vi "Emballage_BDD_Identification_Vdll.vi"(5 "Glissière":refnum<vi>, 6 "lecture seul possible ?":bool, 8 "error in":errorcluster caption="entrée d'erreur", 9 "Posage choisi":string="S112.1229", 11 "chemin connexion complet":path=path "U:/MTD_PRD_TESTS/PARAM_TESTS/PROD_Data-Admin/Support_FAS/Connexion_BDD_VSX.udl") -> (0 "error Out":errorcluster caption="error OUT", 1 "Employe selectionne":T1={"ID Employe"="885", "NOM "="MARTIN SEBASTIEN", "Code ID Employe"="0f00b6435b", "abreviation"="SMA"}, 2 "OK":bool, 3 "lecture seul":bool, 7 "Annulé":bool)   [LabVIEW 2020]
doc: "Vi qui identifie l'utilisateur. Ensuite il vérifie qu'il a ouvert une gamme de travail et finalement qu'il a les accès nécessaire pour ce travail."
uses:
  <vilib>/Utility/error.llb/DialogType.ctl
  Modules/FS/60_FS_Controles/60_FS_SetGet.ctl
panel:
  out "Glissière 2":u8(slide)=100 caption="Identification terminé." scale=0.0..100.0
  out "Table":string[][](table)=[["Nom", "Abréviation", "code", "code bar", "Saisi des H", "Responsable", "S112.1108b", "S112.1065", "S112.1066", "S121.0017", "S122.0009", "Flatprop", "Emballage", "S112.1229/S112.1254", "S112.1289", "S002.0002"], ["YURDAKUL ARZU", "AYU", "AYU_FAS", "0f00b69799", "0", "0", "0", "0", "0", "0", "0", "0", "0", "", "", ""], ["DEDERDING BRIGITTE", "BDE", "BDE_FAS", "0f00b64582", "1", "resp", "1", "1", "1", "1", "1", "1", "1", "1", "1", "1"], ["DA FONSECA CARLOS MANUEL", "CDA", "CDA_FAS", "0f00b64d63", "1", "resp", "1", "1", "1", "1", "1", "1", "1", "1", "1", "1"], ["DOS ANJOS MARIA  CRISTINA", "MDO", "MDO_FAS", "0f00dfc69b", "1", "0", "1", "1", "1", "1", "1", "1", "1", "1", "1", "1"], ["BIANCANIELLO MARIE-JOSE", "MJB", "MJB_FAS", "0f00b65673", "1", "0", "0", "0", "0", "0", "0", "0", "1", "", "", ""], ["DERIVAZ PASCAL", "PDE", "PDE_FAS", "0f00b64c64", "0", "resp", "1", "1", "1", "1", "1", "1", "1", "1", "1", "1"], ["CRAUSAZ-DEMIRTAS SERAP", "SCR", "SCR_FAS", "0f00b64e53", "1", "0", "0", "1", "1", "1", "1", "1", "1", "", "", ""], ["GILLIERON  SABINE", "SLE", "SLE_FAS", "0f00b62fc0", "1", "0", "0", "1", "1", "1", "1", "0", "1", "", "", ""], ["MARTIN SEBASTIEN", "SMA", "SMA_FAS", "0f00b6435b", "1", "resp", "1", "1", "1", "1", "1", "1", "1", "1", "1", "1"], ["VUONG VAN-THANH", "VVT", "VVT_FAS", "0f00b6a8bc", "1", "0", "0", "0", "0", "0", "0", "0", "1", "", "", ""], ["PEREIRA CARLA SOFIA", "PCR", "PCR_FAS", "0f00dfcec4", "1", "0", "0", "0", "0", "0", "0", "1", "1", "", "", ""], ["SANTOS ARMINDA", "ASA", "ASA_FAS", "0f00dfded8", "1", "0", "0", "1", "1", "0", "0", "0", "1", "", "", ""], ["AMANAKO KIBEYA", "KAM", "KAM_FAS", "0f00b6461f", "1", "0", "0", "0", "0", "0", "0", "0", "1", "", "", ""], ["PICOT BRUNO", "BPI", "BPI_FAS", "", "0", "resp", "0", "0", "0", "0", "0", "1", "1", "", "", ""], ["inconnu", "ACK", "ACK_FAS", "inconnu", "0", "resp", "0", "0", "0", "0", "0", "1", "1", "", "", ""], ["FRANCISCO HELIA", "HFR", "HFR_FAS", "0f00ff3428", "1", "0", "0", "1", "1", "0", "0", "0", "1", "", "", ""], ["BERTHOLET MAGALI", "MBE", "MBE_FAS", "0f00debcbf", "1", "0", "0", "0", "0", "0", "0", "1", "1", "", "", ""], ["BEN AYAD DIECKMANN LATIFA", "LBA", "LBA_FAS", "0f00ff602d", "1", "0", "0", "0", "0", "0", "0", "0", "1", "", "", ""], ["ROBERT FABIEN", "FAR", "FAR_FAS", "0f00b648bf", "1", "0", "0", "0", "0", "0", "0", "1", "1", "", "", ""], ["GABRIEL CASSAB SUSANA", "SUG", "SUG_FAS", "0f00b65355", "1", "0", "0", "0", "0", "0", "0", "0", "1", "", "", ""], ["BOURAOUI MOURAD", "MBU", "MBU_FAS", "", "0", "resp", "0", "0", "0", "0", "0", "0", "0", "", "", ""], ["BIGLER ORNELLA", "OBI", "OBI_FAS", "0f00b651a2", "1", "0", "1", "1", "1", "1", "1", "0", "1", "1", "1", "1"], ["BRISSONNETTE MIRELLA", "MBI", "MBI_FAS", "0f00e3ba9c", "1", "0", "0", "0", "0", "0", "0", "1", "1", "", "", ""], ["MARTINS ELISA", "ELM", "ELM_FAS", "0f00debd53", "1", "0", "0", "0", "0", "0", "0", "0", "1", "1", "", ""], ["JEANDENANT PASCALE", "PJE", "PJE_FAS", "0f00ff2670", "1", "0", "0", "0", "0", "0", "0", "0", "1", "", "", ""], ["NECHYTAYLO DARYNA", "DNE", "DNE_FAS", "0f00ff68ed", "1", "0", "0", "0", "0", "0", "0", "1", "1", "", "", ""], ["SILVA MONTEIRO DULCELINA", "DSI", "DSI_FAS", "0f00ff4204", "1", "0", "0", "0", "0", "0", "0", "1", "1", "", "", ""], ["PAHUD ELIANE", "EPU", "EPA_FAS", "0f00ff65d6", "1", "0", "0", "0", "0", "0", "0", "1", "1", "", "", ""], ["THOMASSIN CATHERINE", "TCA", "TCA_FAS", "0f00ff696c", "1", "resp", "0", "0", "0", "0", "0", "0", "0", "1", "1", "1"], ["SIMOND DANIELE", "SDA", "SDA_FAS", "0f00ff2ff9", "1", "0", "0", "0", "0", "0", "0", "0", "0", "", "", ""], ["HORTER VALERIE", "VHO", "VHO_FAS", "0f00ff1ecc", "1", "0", "0", "0", "0", "0", "0", "1", "1", "", "", ""], ["CHENAL JEROME", "JCH", "JCH_FAS", "0f00f6d812", "0", "0", "0", "0", "0", "0", "0", "0", "0", "", "", ""], ["BEN AYAD DIECKMANN LATIFA", "LBA", "LBA_FAS", "0f00ff602d", "1", "0", "0", "0", "0", "0", "0", "0", "0", "", "", ""], ["ANTUNES CARLA MARIA", "CAN", "CAN_FAS", "0f00f76887", "1", "0", "0", "0", "0", "0", "0", "0", "0", "", "", ""], ["DEMIRALMAZ SEMRA", "SDM", "SDM_FAS", "0f00ff42a4", "1", "0", "0", "0", "0", "0", "0", "0", "0", "", "", ""], ["DESARZENS MARIANNE", "MDN", "MDN_FAS", "0f00f6e3b5", "1", "0", "0", "0", "0", "0", "0", "0", "0", "", "", ""], ["inconnu", "HRO", "HRO_FAS", "inconnu", "0", "0", "0", "0", "0", "0", "0", "0", "0", "", "", ""], ["SEMEDO SANCHES MARIA FATIMA", "MSM", "MSM_FAS", "0f00f767ff", "1", "0", "0", "0", "0", "0", "0", "1", "1", "", "", ""], ["inconnu", "PHG", "PHG_FAS", "inconnu", "1", "resp", "1", "1", "1", "1", "1", "1", "1", "1", "1", "1"], ["GUIDEZ LIONEL", "LGU", "LGU_FAS", "0f00f6cad9", "1", "resp", "1", "1", "1", "1", "1", "1", "1", "1", "1", "1"], ["NEVEU CELINE", "CNE", "CNE_FAS", "0f00ff1822", "1", "0", "0", "0", "0", "0", "0", "1", "1", "", "", ""], ["AISSAOUI SAOUSSEN", "SAI", "SAI_FAS", "0f00ff4123", "1", "0", "0", "0", "0", "0", "0", "1", "1", "", "", ""]]
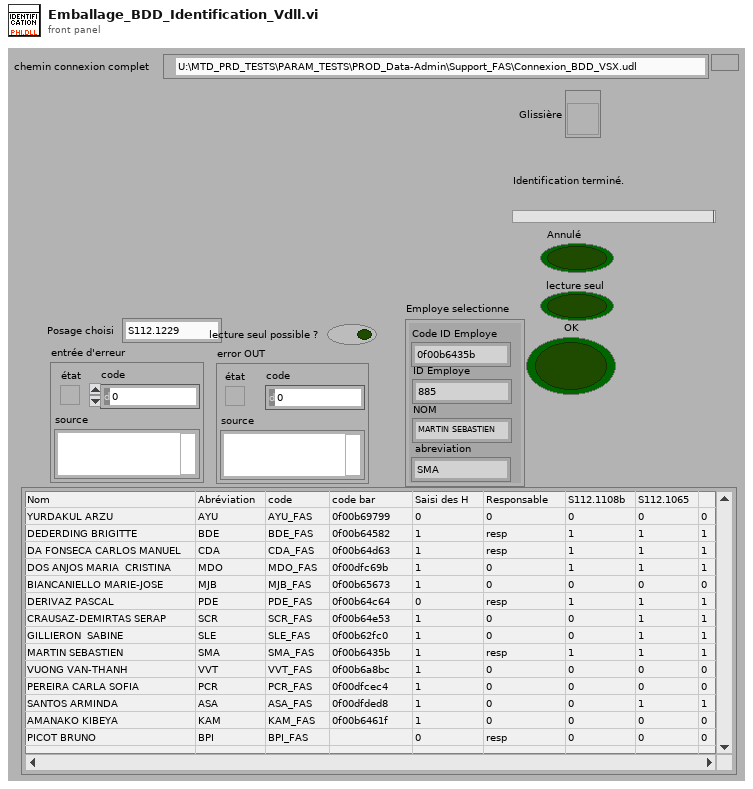
[diagram p1: front panel]
types:
  T1 = cluster{"ID Employe":string, "NOM ":string, "Code ID Employe":string, "abreviation":string}
  T2 = typedef "60_FS_SetGet.ctl" = enum16{"set", "get"}
  T3 = typedef "DialogType.ctl" = u16
  T4 = cluster{"Admin-réseau":path, "XML-Réseau":path, " Résultat tests-Réseau":path, " Archive prôbleme-Réseau":path, " Archive Test  Local":path}
  T5 = cluster{"ID EMPLOYE":string[], "NOM Employé":string[], "Code ID Employé":string[], "abreviation":string[]}
  T6 = typedef "Données employées.ctl" = cluster{"ID heure emp":string, "ID employé":string, "ID ILOT":string, "DATE DEBUT":string, "DATE FIN":string, "Type presence":string, "Remarque":string}
  T7 = cluster{"ID ILOT":string, "ILOT":string, "Departement":string, "Gamme":string}[]
  T8 = typedef "Table type de travail.ctl" = cluster{"LIBELLE":string, "CODE":string, "Remarque":bool}[]
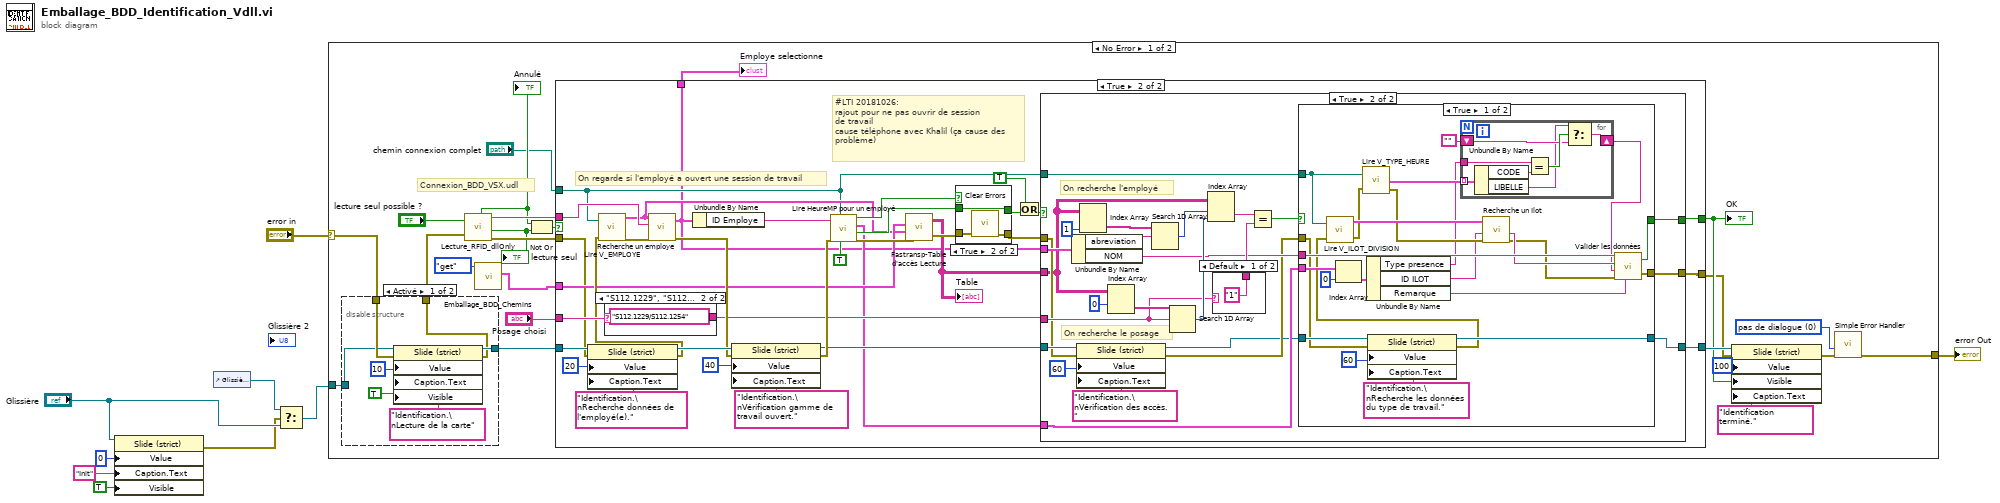
[diagram p0: block diagram]
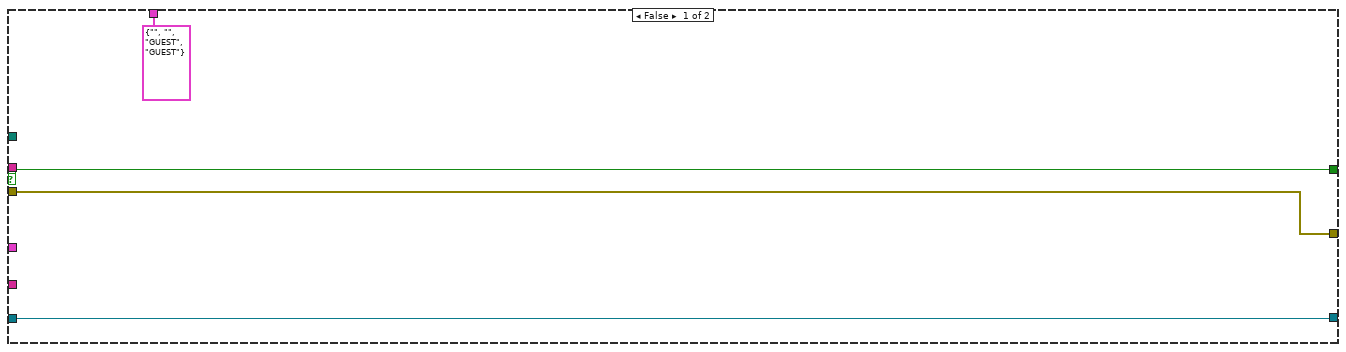
[diagram p3: hidden frame]
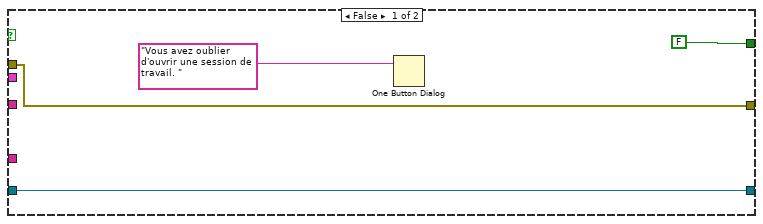
[diagram p4: hidden frame]
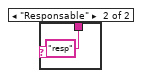
[diagram p5: hidden frame]
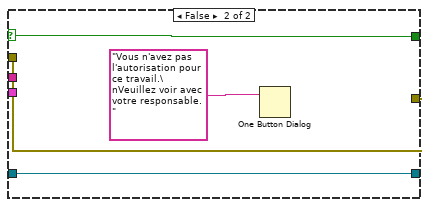
[diagram p6: hidden frame]
diagram:
  n1 = property class="Slide (strict)"(reference="Glissière", "Value"=u8 0, "Caption.Text"="Init", "Visible"=TRUE) -> (error out=w4:errorcluster)  [unwired: 1 in, 1 out]
  n2 = control-ref of="Glissière 2"() -> (w7:refnum<vi>)
  n3 = Select(t=w7, s=w4, f="Glissière") -> (s? t:f=w6:refnum<vi>)
  n4 = case shown="No Error" "error in" {
    selector: "error in" -> [w29 w152]
    tunnel: [w24 w152] -> w8
    tunnel: w6 -> [w13 _]
    frame No Error {
      w15 = T3 0 items=["pas de dialogue", "Message OK", "Message continuer ou arrêter", "Message OK + mises en garde", "Arrêter/Continuer + mises en garde"] ("type of dialog (OK msg:1)")
      # "Connexion_BDD_VSX.udl"
      n5 = disable-structure shown="Activé" {
        disable-tunnel: [w37 _] -> w30
        disable-tunnel: w29 -> [w36 w40]
        disable-tunnel: [w34 w40] -> w16
        disable-tunnel: w13 -> [w33 _]
        frame Enabled {
          n6 = property class="Slide (strict)"(reference=w33, error in=w36, "Value"=u8 10 ("Valeur"), "Caption.Text"="Identification.\nLecture de la carte" ("Sous-titre.Texte"), "Visible"=TRUE) -> (reference out=w37:refnum<vi>, error out=w34:errorcluster)
        }
        frame Disabled {
        }
      }
      n7 = call "Lecture_RFID_dllOnly .vi"("error in"=w16, "lecture seul possible ?"="lecture seul possible ?") -> ("error out"=w32:errorcluster, "lecture seul"=w20:bool, "Code Employe"=w31:string, "Annulé"=w18:bool)  [unwired: 1 out]
      "Annulé" <- w18
      "lecture seul" <- w20
      n8 = call "Emballage_BDD_Chemins.vi"("SetGet"=60_FS_SetGet."get") -> ("CLT_Chemins_out"=w11:T4)  [unwired: 9 in, 1 out]
      n9 = Not Or(1:w20, 2:w18) -> (0:w19:bool)
      n10 = case shown="True" w19 {
        selector: w19 -> [w44 _]
        tunnel: w32 -> [w43 w58]
        tunnel: w31 -> [_ w78]
        tunnel: "chemin connexion complet" -> [_ w49]
        tunnel: "Posage choisi" -> [_ w73]
        tunnel: [w44 w77] -> w26
        tunnel: [w43 w76] -> w23
        tunnel: w11 -> [_ w62]
        tunnel: w30 -> [w42 w68]
        tunnel: [w42 w60] -> w28
        tunnel: [T1 {"ID Employe"="", "NOM "="", "Code ID Employe"="GUEST", "abreviation"="GUEST"} ("Employe selectionne") w48] -> w17
        frame False {
        }
        frame True {
          # "#LTI 20181026:\nrajout pour ne pas ouvrir de session\nde travail\ncause téléphone avec Khalil (ça cause des\nproblème)"
          # "On regarde si l'employé a ouvert une session de travail"
          n11 = property class="Slide (strict)"(reference=w68, error in=w58, "Value"=u8 20 ("Valeur"), "Caption.Text"="Identification.\nRecherche données de l'employé(e)." ("Sous-titre.Texte")) -> (reference out=w67:refnum<vi>, error out=w66:errorcluster)
          n12 = call "Lire V_EMPLOYE.vi"("error in (no error)"=w66, "connection information"=w49) -> ("error out"=w75:errorcluster, "EMPLOYE"=w52:T5)
          n13 = case shown="\"S112.1229\", \"S112.1254\"" w73 {
            selector: w73 -> [w150 _]
            tunnel: [w150 "S112.1229/S112.1254"] -> w59
            frame Default {
            }
            frame "S112.1229", "S112.1254" {
            }
          }
          n14 = call "Recherche un employe.vi"("EMPLOYE"=w52, "Code ID Employe"=w78, "error in"=w75) -> ("Employe selectionne"=w48:T1, "error out"=w65:errorcluster)  [unwired: 2 in]
          n15 = Unbundle By Name(w48) -> ("ID Employe"=w74:string)
          n16 = property class="Slide (strict)"(reference=w67, error in=w65, "Value"=u8 40 ("Valeur"), "Caption.Text"="Identification.\nVérification gamme de travail ouvert." ("Sous-titre.Texte")) -> (reference out=w61:refnum<vi>, error out=w64:errorcluster)
          n17 = call "Lire HeureMP pour un employé.vi"("sans fin ?"=TRUE, "connection information"=w49, "error in"=w64, "ID employe"=w74) -> ("error out"=w63:errorcluster, "existe ?"=w54:bool, "HeureMP employé"=w50:T6[], "Erreur de\n comunication"=w55:bool)  [unwired: 2 in, 1 out]
          n18 = call "Fastransp-Table d'accès Lecture.vi"("error in"=w63, "EMPLOYE"=w52, "Chemin"=w62) -> ("error out"=w57:errorcluster, "Table"=w51:string[][])  [unwired: 1 in]
          "Table" <- w51
          n19 = case shown="True" w55 {
            tunnel: w57 -> [w146 w149]
            tunnel: [w146 w148] -> w56
            tunnel: w54 -> [w145 w147]
            tunnel: [w145 w147] -> w47
            frame False {
            }
            frame True {
              n20 = call <vilib>:"Clear Errors.vi"("error in (no error)"=w149) -> ("error out"=w148:errorcluster)  [unwired: 5 in, 1 out]
            }
          }
          n21 = Or(x=TRUE, y=w47) -> (x .or. y?=w46:bool)
          n22 = case shown="True" w46 {
            tunnel: w48 -> [_ w107]
            tunnel: [FALSE ("refuser les données") w106] -> w77
            tunnel: [w80 w105] -> w76
            tunnel: w61 -> [w82 w90]
            tunnel: [w82 w83] -> w60
            tunnel: w59 -> [_ w89]
            tunnel: w56 -> [w80 w88]
            tunnel: w51 -> [_ w87]
            tunnel: w50 -> [_ w86]
            tunnel: w49 -> [_ w85]
            frame False {
              n23 = One Button Dialog(message="Vous avez oublier d'ouvrir une session de travail. ") -> ()  [unwired: 1 in, 1 out]
            }
            frame True {
              # "On recherche le posage"
              # "On recherche l'employé"
              n24 = Unbundle By Name(w107) -> ("abreviation"=w100:string, "NOM"=w94:string)
              n25 = property class="Slide (strict)"(reference=w90, error in=w88, "Value"=u8 60 ("Valeur"), "Caption.Text"="Identification.\nVérification des accès." ("Sous-titre.Texte")) -> (reference out=w84:refnum<vi>, error out=w91:errorcluster)
              n26 = Index Array(array=w87, index (col)=1 ("indice désactivé (col)")) -> (element=w102:string[])  [unwired: 1 in]
              n27 = Index Array(array=w87, index (row)=0 ("indice (ligne)")) -> (element=w96:string[])  [unwired: 1 in]
              n28 = Search 1D Array(1D array=w102, element=w100) -> (index of element=w103:i32)  [unwired: 1 in]
              n29 = Search 1D Array(1D array=w96, element=w89) -> (index of element=w99:i32)  [unwired: 1 in]
              n30 = Index Array(array=w87, index (row)=w103, index (col)=w99) -> (element=w104:string)
              n31 = case shown="Default" w89 {
                tunnel: ["1" ("y") "resp" ("y")] -> w95
                frame Default {
                }
                frame "Responsable" {
                }
              }
              n32 = Equal?(x=w104, y=w95) -> (x = y?=w98:bool)
              n33 = case shown="True" w98 {
                selector: w98 -> [_ w143]
                tunnel: [w128 w143] -> w106
                tunnel: w94 -> [w133 _]
                tunnel: w91 -> [w111 w142]
                tunnel: [w129 w142] -> w105
                tunnel: w86 -> [w132 _]
                tunnel: w85 -> [w125 _]
                tunnel: w84 -> [w113 w141]
                tunnel: [w112 w141] -> w83
                frame True {
                  n34 = Index Array(array=w132, index=0 ("indice")) -> (element=w130:T6)
                  n35 = Unbundle By Name(w130) -> ("Type presence"=w119:string, "ID ILOT"=w120:string, "Remarque"=w117:string)
                  n36 = property class="Slide (strict)"(reference=w113, error in=w111, "Value"=u8 60 ("Valeur"), "Caption.Text"="Identification.\nRecherche les données du type de travail." ("Sous-titre.Texte")) -> (reference out=w112:refnum<vi>, error out=w110:errorcluster)
                  n37 = call "Lire V_ILOT_DIVISION.vi"("error in"=w110, "connection information"=w125) -> ("error out"=w122:errorcluster, "Table Ilot-Dep-Gamme"=w127:T7)
                  n38 = call "Lire V_TYPE_HEURE.vi"("connection information"=w125, "error in"=w122) -> ("Table type travail"=w123:T8, "error out"=w121:errorcluster)  [unwired: 1 out]
                  n39 = for {
                    tunnel: w123 -> [w140] mode=indexing
                    tunnel: w119 -> [w138]
                    shift-right: [w136] -> w118
                    shift-left: "" -> [w135]
                    n40 = Unbundle By Name(w140) -> ("CODE"=w139:string, "LIBELLE"=w134:string)
                    n41 = Equal?(x=w138, y=w139) -> (x = y?=w137:bool)
                    n42 = Select(t=w134, s=w137, f=w135) -> (s? t:f=w136:string)
                  }
                  n43 = call "Recherche un Ilot.vi"("Table Gamme-Dep-Ilot IN"=w127, "ID ILOT"=w120, "error in (no error)"=w121) -> ("Gamme-Dep-Ilot"=w126:string, "error out"=w116:errorcluster)  [unwired: 1 in, 3 out]
                  n44 = call "Valider les données.vi"("Employé(e) :"=w133, "Gamme-Dep-Ilot"=w126, "Type de travail :"=w118, "error in"=w116, "Commentaire"=w117) -> ("Validé ?"=w128:bool, "error out"=w129:errorcluster)
                }
                frame False {
                  n45 = One Button Dialog(message="Vous n'avez pas  l'autorisation pour ce travail.\nVeuillez voir avec votre responsable.") -> ()  [unwired: 1 in, 1 out]
                }
              }
            }
          }
        }
      }
      "OK" <- w26
      "Employe selectionne" <- w17
      n46 = property class="Slide (strict)"(reference=w28, error in=w23, "Value"=u8 100 ("Valeur"), "Visible"=w26, "Caption.Text"="Identification terminé." ("Sous-titre.Texte")) -> (error out=w22:errorcluster)  [unwired: 1 out]
      n47 = call <vilib>:"Simple Error Handler.vi"("type of dialog (OK msg:1)"=w15, "error in (no error)"=w22) -> ("error out"=w24:errorcluster)  [unwired: 3 in, 4 out]
    }
    frame Error {
    }
  }
  "error Out" <- w8
